vi "FGV_DOCK_login.vi"(6 "login_refnums":T1, 7 "options":T2, 8 "error_in":errorcluster, 9 "access_level_in":i32, 10 "username_in":string, 11 "ID_in":string) -> (0 "error_out":errorcluster, 1 "access_level_out":i32, 2 "username_out":string, 3 "ID_out":string, 5 "Login read active?":bool)   [LabVIEW 2019]
uses:
  FGV_DOCK_login.ctl
  DOCK_login_refnums.ctl
  controls_state/FGV_DOCK_controls_state.ctl
  DOCK_multistate_indicator/FGV_DOCK_multistate_indicator.ctl
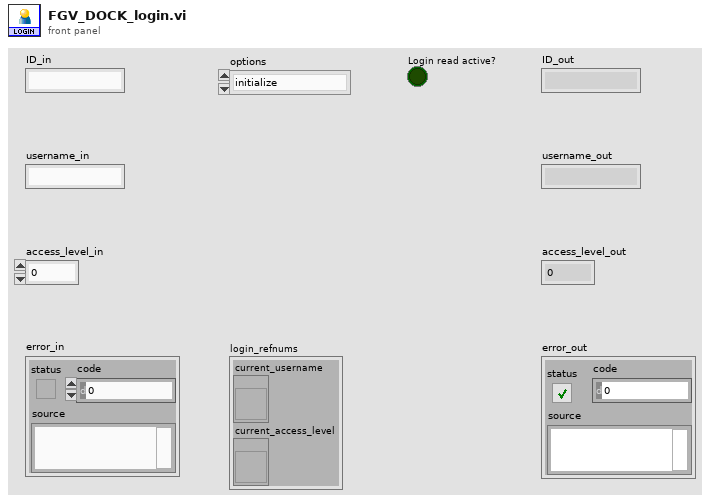
[diagram p1: front panel]
types:
  T1 = typedef "DOCK_login_refnums.ctl" = cluster{"current_username":refnum<vi>, "current_access_level":refnum<vi>}
  T2 = typedef "FGV_DOCK_login.ctl" = enum16{"initialize", "start_login_read", "end_login_read", "login", "logout", "get_login_info"}
  T3 = typedef "FGV_DOCK_controls_state.ctl" = enum16{"initialize", "login_event", "translation_event", "batch_event", "reload_event", "gear_event", "gear_saved_event", "gear_in_another_batch_event", "gear_in_current_batch_event", "NOK_ref_gear_event", "NOK_station_gear_event", "get_gear_loaded_status"}
  T4 = typedef "FGV_DOCK_multistate_indicator.ctl" = enum16{"initialize", "login", "logout", "start_batch", "finish_batch", "gear_OK", "gear_NOK", "gear_clear", "translate", "error", "error_clear"}
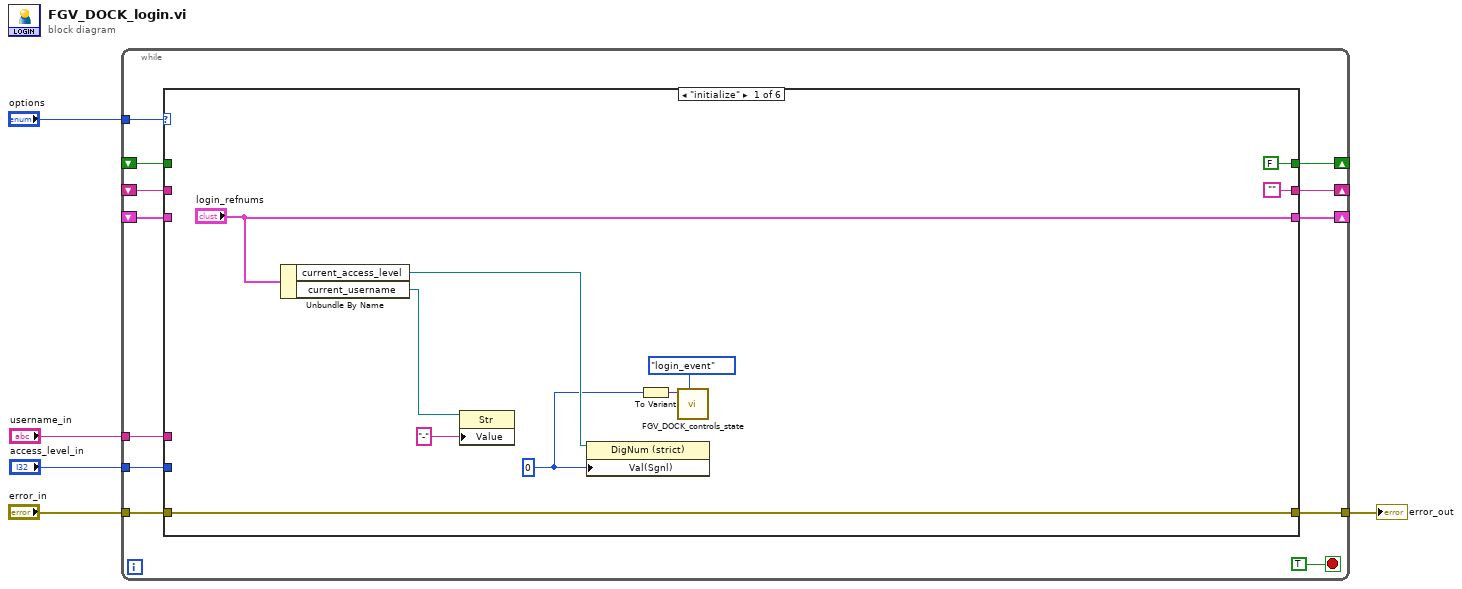
[diagram p0: block diagram]
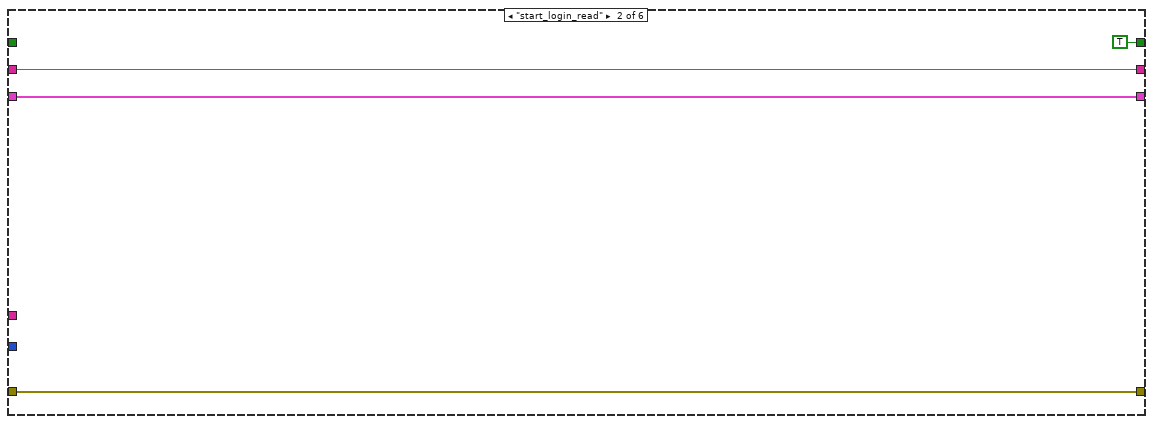
[diagram p2: hidden frame]
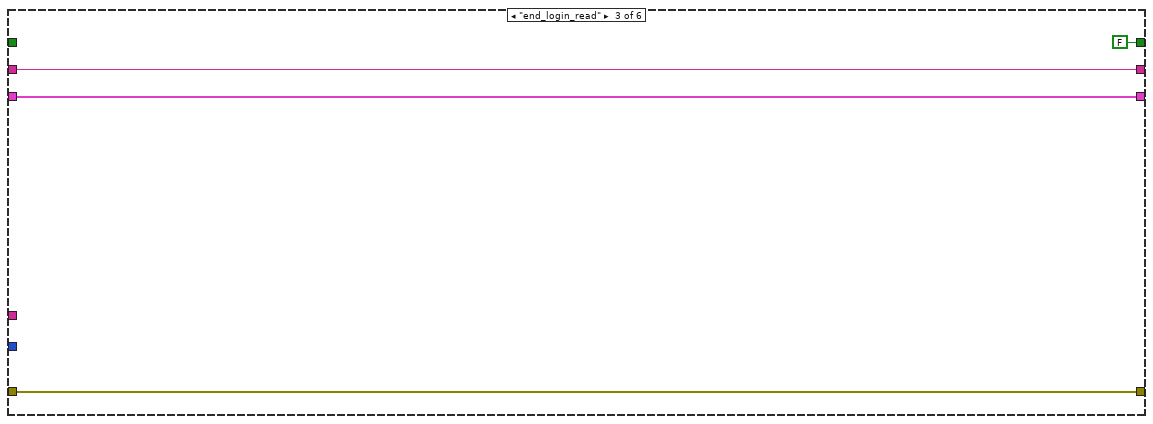
[diagram p3: hidden frame]
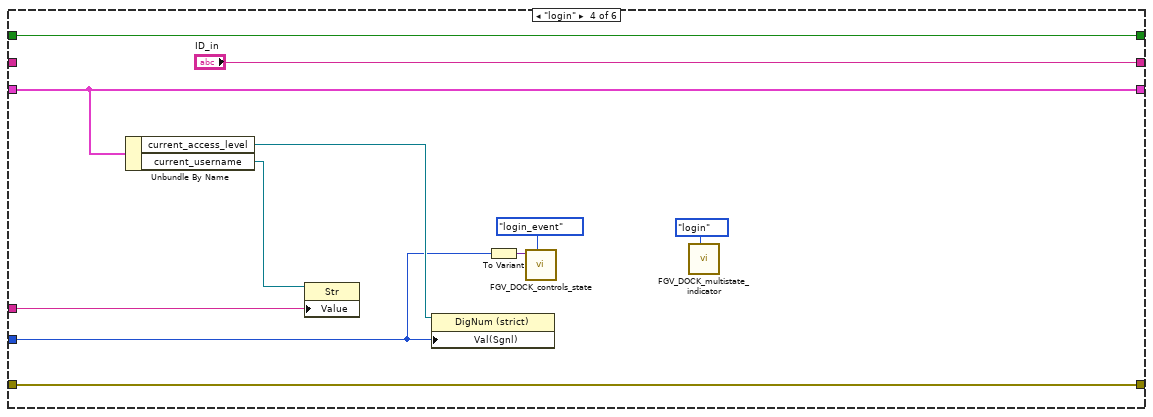
[diagram p4: hidden frame]
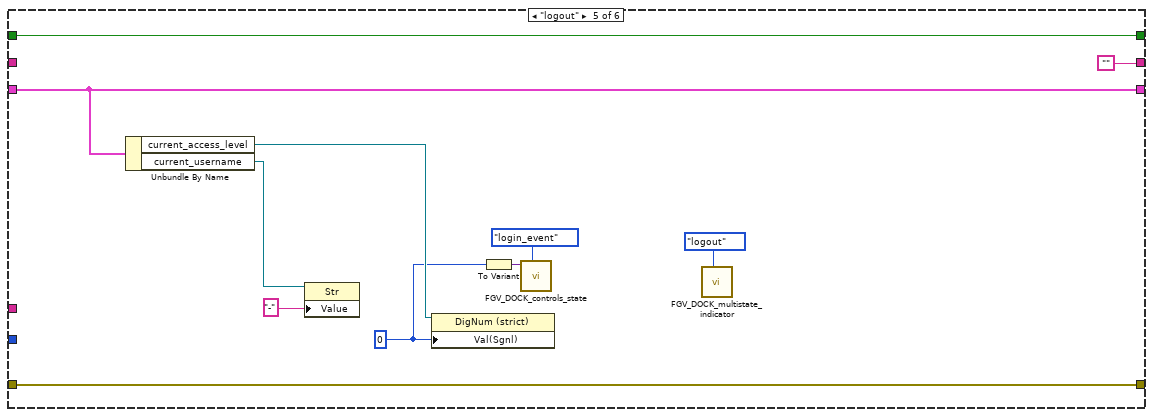
[diagram p5: hidden frame]
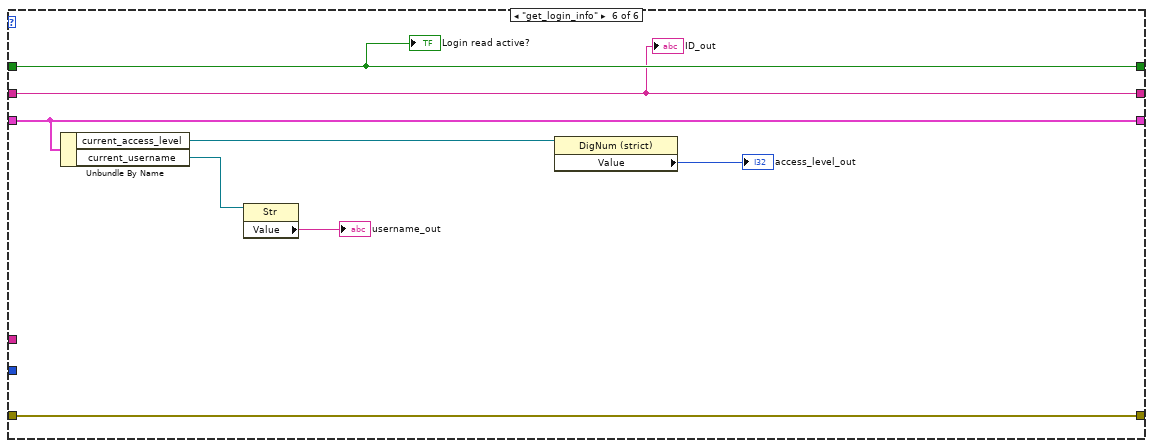
[diagram p6: hidden frame]
diagram:
  n1 = while {
    tunnel: "options" -> [w16]
    tunnel: [w15] -> w5
    tunnel: "error_in" -> [w14]
    shift-right: [w13] -> _
    shift-left: _ -> [w12]
    tunnel: "username_in" -> [w11]
    tunnel: "access_level_in" -> [w10]
    shift-right: [w9] -> _
    shift-left: _ -> [w8]
    shift-right: [w7] -> _
    shift-left: _ -> [w6]
    stop <- TRUE stop-if-true
    n2 = case shown="\"initialize\"" w16 {
      tunnel: [w27 w31 w35 w46 w57 w65] -> w15
      tunnel: w14 -> [w27 w31 w35 w46 w57 w65]
      tunnel: ["login_refnums" w30 w32 w42 w53 w64] -> w13
      tunnel: w12 -> [_ w30 w32 w42 w53 w64]
      tunnel: w11 -> [_ _ _ w45 _ _]
      tunnel: w10 -> [_ _ _ w37 _ _]
      tunnel: ["" w29 w33 "ID_in" "" w58] -> w9
      tunnel: w8 -> [_ w29 w33 _ _ w58]
      tunnel: [FALSE TRUE FALSE w40 w51 w60] -> w7
      tunnel: w6 -> [_ _ _ w40 w51 w60]
      frame "initialize" {
        w18 = 0 ("Value")
        n3 = Unbundle By Name("login_refnums") -> ("current_access_level"=w25:refnum<vi>, "current_username"=w26:refnum<vi>)
        n4 = property class="Str"(reference=w26, "Value"="-") -> ()  [unwired: 1 in, 2 out]
        n5 = property class="DigNum (strict)"(reference=w25, "Val(Sgnl)"=w18) -> ()  [unwired: 1 in, 2 out]
        n6 = To Variant(anything=w18) -> (Variant=w19:variant)
        n7 = call "FGV_DOCK_controls_state.vi"("options"=FGV_DOCK_controls_state."login_event", "input"=w19) -> ()  [unwired: 8 in, 2 out]
      }
      frame "start_login_read" {
      }
      frame "end_login_read" {
      }
      frame "login" {
        n8 = Unbundle By Name(w42) -> ("current_access_level"=w43:refnum<vi>, "current_username"=w44:refnum<vi>)
        n9 = property class="Str"(reference=w44, "Value"=w45) -> ()  [unwired: 1 in, 2 out]
        n10 = property class="DigNum (strict)"(reference=w43, "Val(Sgnl)"=w37) -> ()  [unwired: 1 in, 2 out]
        n11 = To Variant(anything=w37) -> (Variant=w38:variant)
        n12 = call "FGV_DOCK_controls_state.vi"("options"=FGV_DOCK_controls_state."login_event", "input"=w38) -> ()  [unwired: 8 in, 2 out]
        n13 = call "FGV_DOCK_multistate_indicator.vi"("options"=FGV_DOCK_multistate_indicator."login") -> ()  [unwired: 10 in, 1 out]
      }
      frame "logout" {
        w48 = 0 ("Value")
        n14 = Unbundle By Name(w53) -> ("current_access_level"=w55:refnum<vi>, "current_username"=w56:refnum<vi>)
        n15 = property class="Str"(reference=w56, "Value"="-") -> ()  [unwired: 1 in, 2 out]
        n16 = property class="DigNum (strict)"(reference=w55, "Val(Sgnl)"=w48) -> ()  [unwired: 1 in, 2 out]
        n17 = To Variant(anything=w48) -> (Variant=w49:variant)
        n18 = call "FGV_DOCK_controls_state.vi"("options"=FGV_DOCK_controls_state."login_event", "input"=w49) -> ()  [unwired: 8 in, 2 out]
        n19 = call "FGV_DOCK_multistate_indicator.vi"("options"=FGV_DOCK_multistate_indicator."logout") -> ()  [unwired: 10 in, 1 out]
      }
      frame "get_login_info" {
        n20 = Unbundle By Name(w64) -> ("current_access_level"=w62:refnum<vi>, "current_username"=w63:refnum<vi>)
        n21 = property class="Str"(reference=w63) -> ("Value"=→"username_out":string)  [unwired: 1 in, 2 out]
        n22 = property class="DigNum (strict)"(reference=w62) -> ("Value"=→"access_level_out":i32)  [unwired: 1 in, 2 out]
        "Login read active?" <- w60
        "ID_out" <- w58
      }
    }
  }
  "error_out" <- w5
